vi "Virbration ListFGV.vi"(0 "TableIn":string[](array[string])=["Default", "", "", " 0"], 1 "Action":T1(ring)=enum."WrteAll", 7 "Y":i32, 9 "DataIn":string, 11 "error in":errorcluster) -> (4 "TableOut":string[](array[string]), 10 "DataOut":string, 15 "error out":errorcluster)   [LabVIEW 2019]
uses:
  09bdc40f-24f8-42fa-be14-94a5734f4f81.vi
  3a88f7dc-0fdf-4cec-95e5-a4f3429e1c34.vi
  LLB/Commonly VI/Main Glb.vi
  <vilib>/JDP Science/JSONtext/Variant to JSON Text.vi
  <vilib>/JDP Science/JSONtext/JSON text to Variant.vi
  LLB/Commonly VI.lvlib
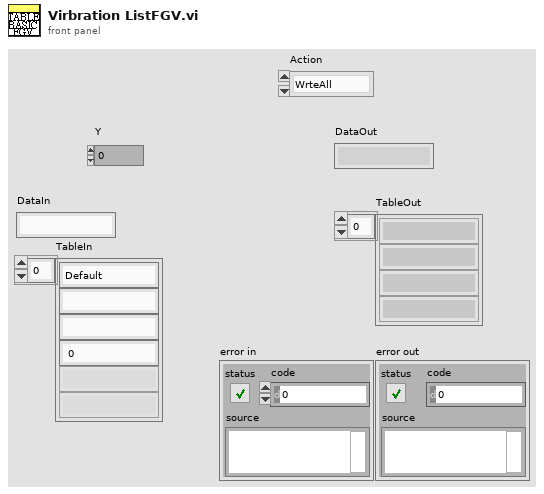
[diagram p1: front panel]
types:
  T1 = enum16{"Initial", "Write", "Read", "Save", "Load", "WrteAll"}
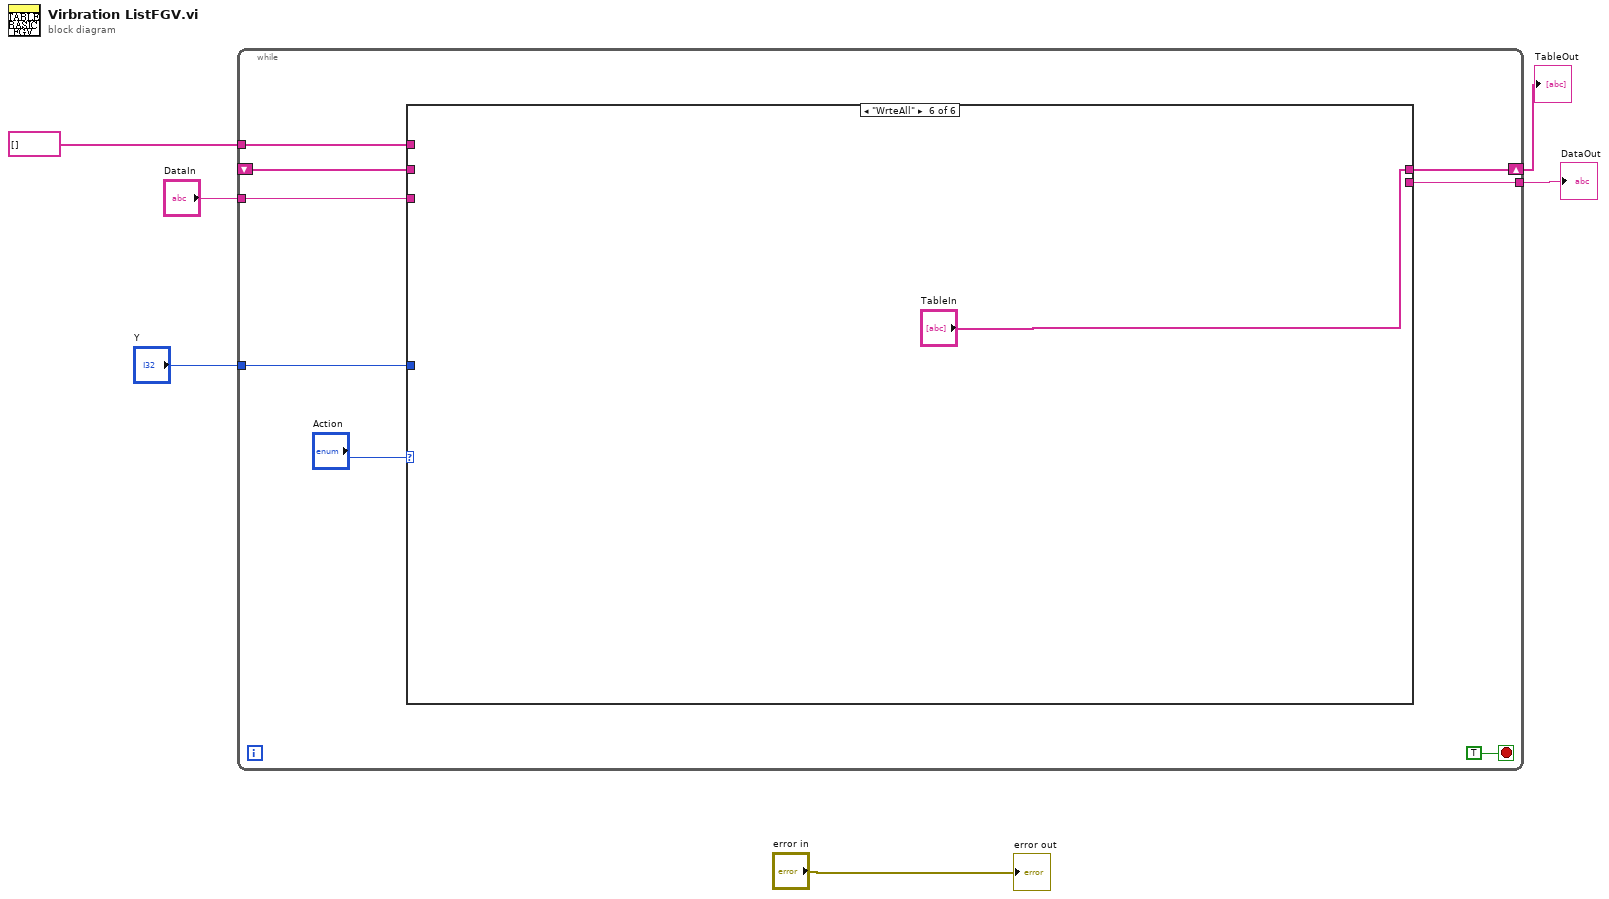
[diagram p0: block diagram]
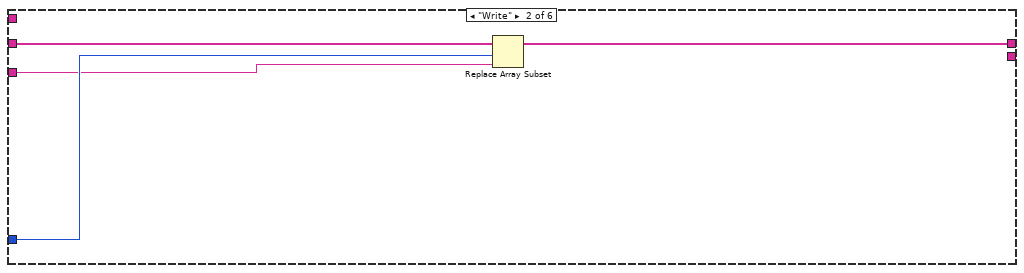
[diagram p3: hidden frame]
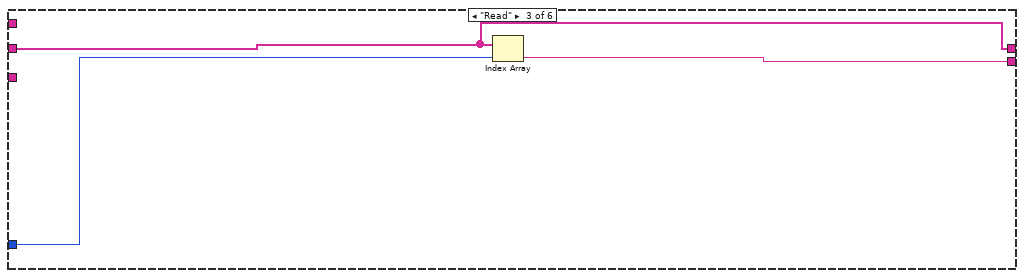
[diagram p4: hidden frame]
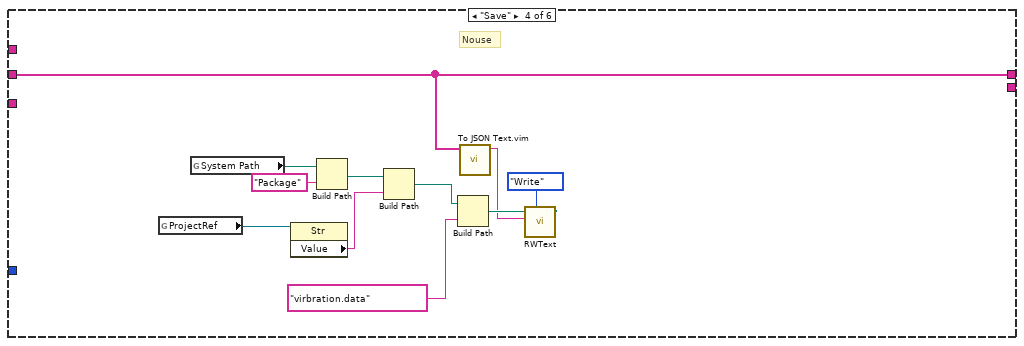
[diagram p5: hidden frame]
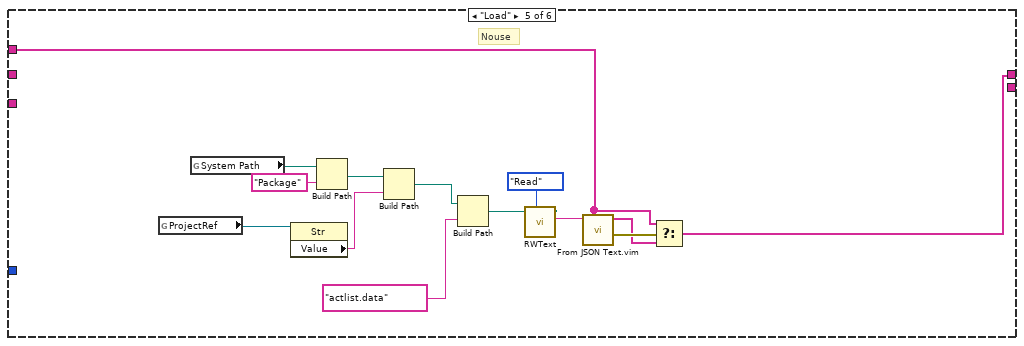
[diagram p6: hidden frame]
diagram:
  n1 = while {
    shift-right: [w14] -> w2
    shift-left: _ -> [w13]
    tunnel: string[] [] ("Item Names") -> [w12]
    tunnel: "Y" -> [w10]
    tunnel: "DataIn" -> [w9]
    tunnel: [w7] -> w5
    stop <- TRUE stop-if-true
    n2 = case shown="\"WrteAll\"" "Action" {
      tunnel: [w15 w19 w21 w24 w34 "TableIn"] -> w14
      tunnel: w13 -> [_ w18 w21 w24 _ _]
      tunnel: w12 -> [w15 _ _ _ w36 _]
      tunnel: w10 -> [_ w17 w22 _ _ _]
      tunnel: w9 -> [_ w16 _ _ _ _]
      tunnel: [_ _ w20 _ _ _] -> w7
      frame "Initial", Default {
      }
      frame "Write" {
        n3 = Replace Array Subset(array=w18, new element=w16, index=w17) -> (w19:string[])
      }
      frame "Read" {
        n4 = Index Array(array=w21, index=w22) -> (element=w20:string)
      }
      frame "Save" {
        # "Nouse"
        n5 = global read "Main Glb.vi" "ProjectRef"() -> (w30:refnum<vi>)
        n6 = global read "Main Glb.vi" "System Path"() -> (w33:path)
        n7 = property class="Str"(reference=w30) -> ("Value"=w29:string)  [unwired: 1 in, 2 out]
        n8 = Build Path(base path=w33, name or relative path="Package") -> (appended path=w31:path)
        n9 = Build Path(base path=w31, name or relative path=w29) -> (appended path=w27:path)
        n10 = Build Path(base path=w27, name or relative path="virbration.data") -> (appended path=w25:path)
        n11 = call "To JSON Text.vim"("Anything"=w24) -> ("<JSON>"=w23:string)  [unwired: 9 in, 1 out]
        n12 = call "RWText.vi"("Action"=enum16{"Read", "Write"}."Write", "TextIn"=w23, "file path (use dialog)"=w25) -> ()  [unwired: 7 in, 2 out]
      }
      frame "Load" {
        # "Nouse"
        n13 = global read "Main Glb.vi" "ProjectRef"() -> (w44:refnum<vi>)
        n14 = global read "Main Glb.vi" "System Path"() -> (w47:path)
        n15 = property class="Str"(reference=w44) -> ("Value"=w43:string)  [unwired: 1 in, 2 out]
        n16 = Build Path(base path=w47, name or relative path="Package") -> (appended path=w45:path)
        n17 = Build Path(base path=w45, name or relative path=w43) -> (appended path=w41:path)
        n18 = Build Path(base path=w41, name or relative path="actlist.data") -> (appended path=w39:path)
        n19 = call "RWText.vi"("Action"=enum16{"Read", "Write"}."Read", "file path (use dialog)"=w39) -> ("textOut"=w38:string)  [unwired: 8 in, 1 out]
        n20 = call "From JSON Text.vim"("Data Type and Default Value"=w36, "JSON"=w38) -> ("error out"=w37:errorcluster, "Data out"=w35:string[])  [unwired: 8 in]
        n21 = Select(t=w36, s=w37, f=w35) -> (s? t:f=w34:string[])
      }
      frame "WrteAll" {
      }
    }
  }
  "DataOut" <- w5
  "TableOut" <- w2
  "error out" <- "error in"
